vi "Measurement Logic.vi"() -> ()   [LabVIEW 2021, in "Ripple_PMIC.lvlib"]
uses:
  Ripple_PMIC.lvlib
  <vilib>/MeasurementLink/MeasurementLink Measurement Server/Measure Call Context/Measure Call Context.lvclass
  Measurement Results.ctl
  Measurement Configuration.ctl
  <instrlib>/niDCPower/nidcpower.llb/niDCPower Output Function.ctl
  <instrlib>/niDCPower/nidcpower.llb/niDCPower Sense.ctl
  <instrlib>/niDCPower/nidcpower.llb/niDCPower Source Mode.ctl
  <instrlib>/niDCPower/nidcpower.llb/niDCPower Wait For Event - Event.ctl
  <instrlib>/niDCPower/nidcpower.llb/niDCPower Measurement Type.ctl
  <instrlib>/niScope/Controls/niScope vertical coupling.ctl
  <instrlib>/niScope/Controls/niScope trigger slope.ctl
  <instrlib>/niScope/Controls/niScope trigger coupling.ctl
  <instrlib>/niScope/Configure/Trigger/niScope Configure Trigger Edge.vi
  <vilib>/MeasurementLink/MeasurementLink Measurement Server/Measure Call Context/Accessor/Is Canceled.vi
  <instrlib>/niDCPower/nidcpower.llb/niDCPower Get Channel Name From String.vi
  <instrlib>/niScope/Controls/niScope timestamp type.ctl
  <vilib>/measure/NI_MAPro.lvlib
  <vilib>/measure/madcrms.llb/Basic Averaged DC-RMS for 1 Chan.vi
  <instrlib>/niScope/Acquire/Fetch/niScope Fetch WDT.vi
panel:
  in  "measurement configuration":T1={"Mode of operation"=enum."Perform measurement", "Source resource name"="", "Source voltage level"=10.0, "Source current limit"=15.0, "Load resource name"="", "Load current level"=6.0, "Load voltage limit range"=6.0, "Scope resource name"="", "Scope channel name"="0", "Scope sample rate"=10000.0, "Scope acquisition time"=3.0, "Scope probe attenuation"=1.0}
  out "measurement results":T2
  out "measure call context out":refnum<class "Measure Call Context.lvclass">
  in  "measure call context in":refnum<class "Measure Call Context.lvclass">
  out "error out":errorcluster
  in  "error in":errorcluster
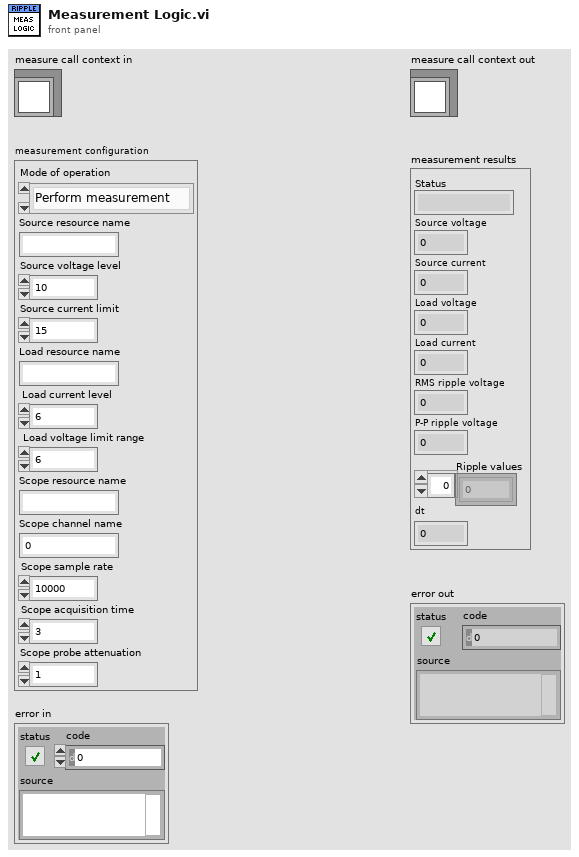
[diagram p1: front panel]
types:
  T1 = typedef "Ripple_PMIC.lvlib/Measurement Configuration.ctl" = cluster{"Mode of operation":enum32{"Power on the DUT", "Perform measurement", "Power off the DUT"}, "Source resource name":string, "Source voltage level":dbl, "Source current limit":dbl, "Load resource name":string, "Load current level":dbl, "Load voltage limit range":dbl, "Scope resource name":string, "Scope channel name":string, "Scope sample rate":dbl, "Scope acquisition time":dbl, "Scope probe attenuation":dbl}
  T2 = typedef "Ripple_PMIC.lvlib/Measurement Results.ctl" = cluster{"Status":string, "Source voltage":dbl, "Source current":dbl, "Load voltage":dbl, "Load current":dbl, "RMS ripple voltage":dbl, "P-P ripple voltage":dbl, "Ripple values":dbl[], "dt":dbl}
  T3 = cluster{"Source Session":refnum<k15>, "Load Session":refnum<k15>, "Scope Session":refnum<k15>, "Source channel":string, "Load channel":string}
  T4 = enum32{"Power on the DUT", "Perform measurement", "Power off the DUT"}
  T5 = typedef "niDCPower Wait For Event - Event.ctl" = i32
  T6 = typedef "niDCPower Source Mode.ctl" = i32
  T7 = typedef "niDCPower Sense.ctl" = i32
  T8 = typedef "niDCPower Output Function.ctl" = i32
  T9 = typedef "niDCPower Measurement Type.ctl" = i32
  T10 = typedef "niScope trigger coupling.ctl" = u16
  T11 = typedef "niScope trigger slope.ctl" = i32
  T12 = typedef "niScope vertical coupling.ctl" = i32
  T13 = typedef "niScope timestamp type.ctl" = i32
  T14 = cluster{"actualSamples":i32, "absoluteInitialX":dbl, "relativeInitialX":dbl, "xIncrement":dbl, "offset":dbl, "gain":dbl, "reserved1":dbl, "reserved2":dbl}
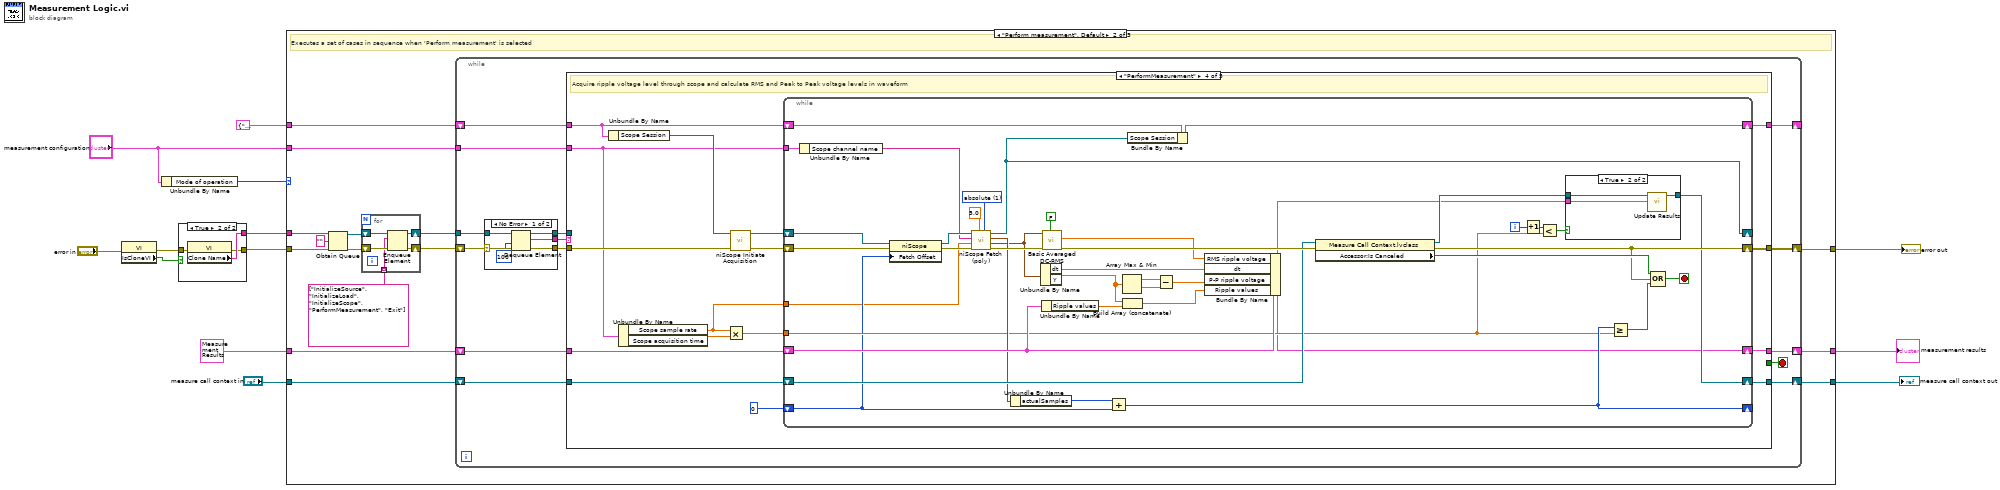
[diagram p0: block diagram]
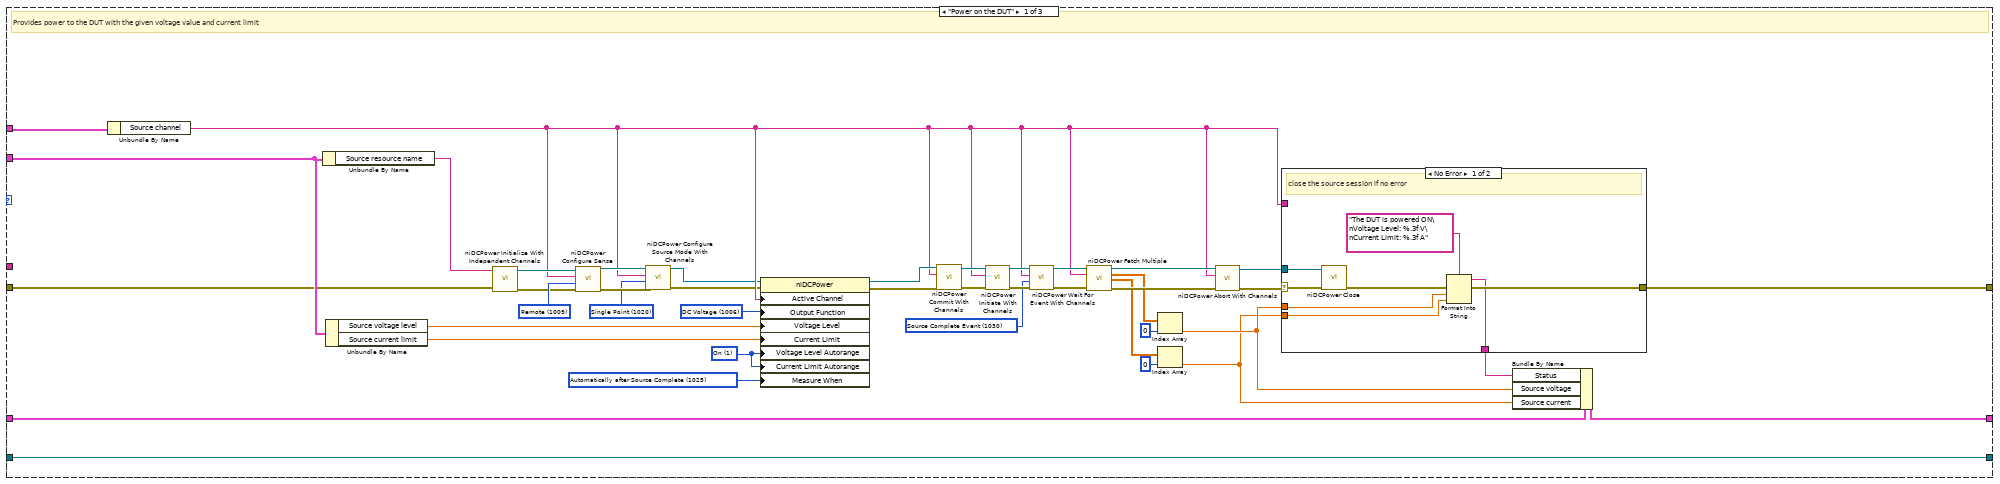
[diagram p2: hidden frame]
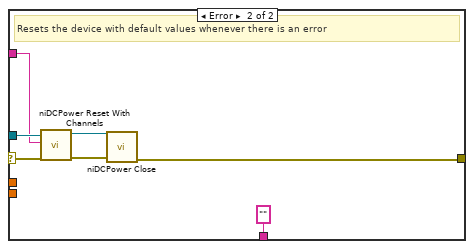
[diagram p3: hidden frame]
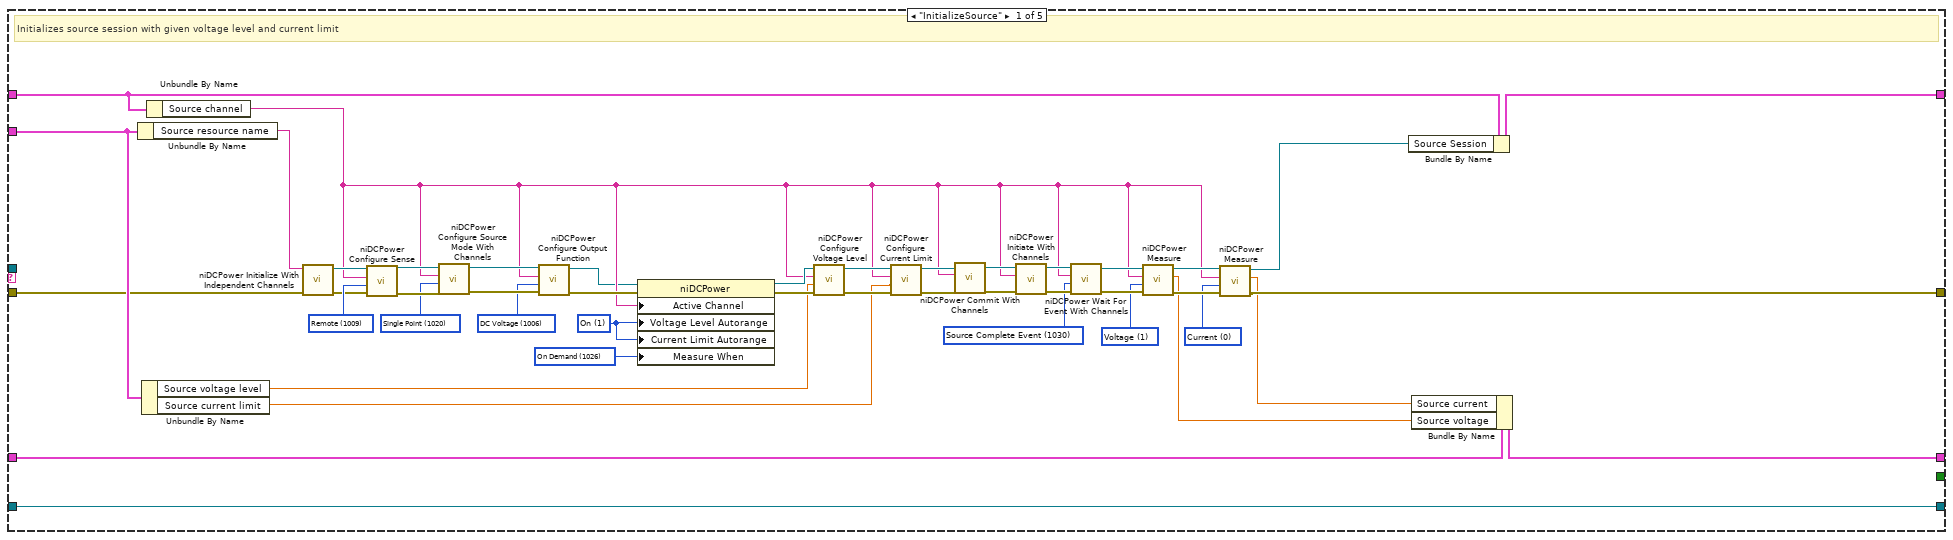
[diagram p4: hidden frame]
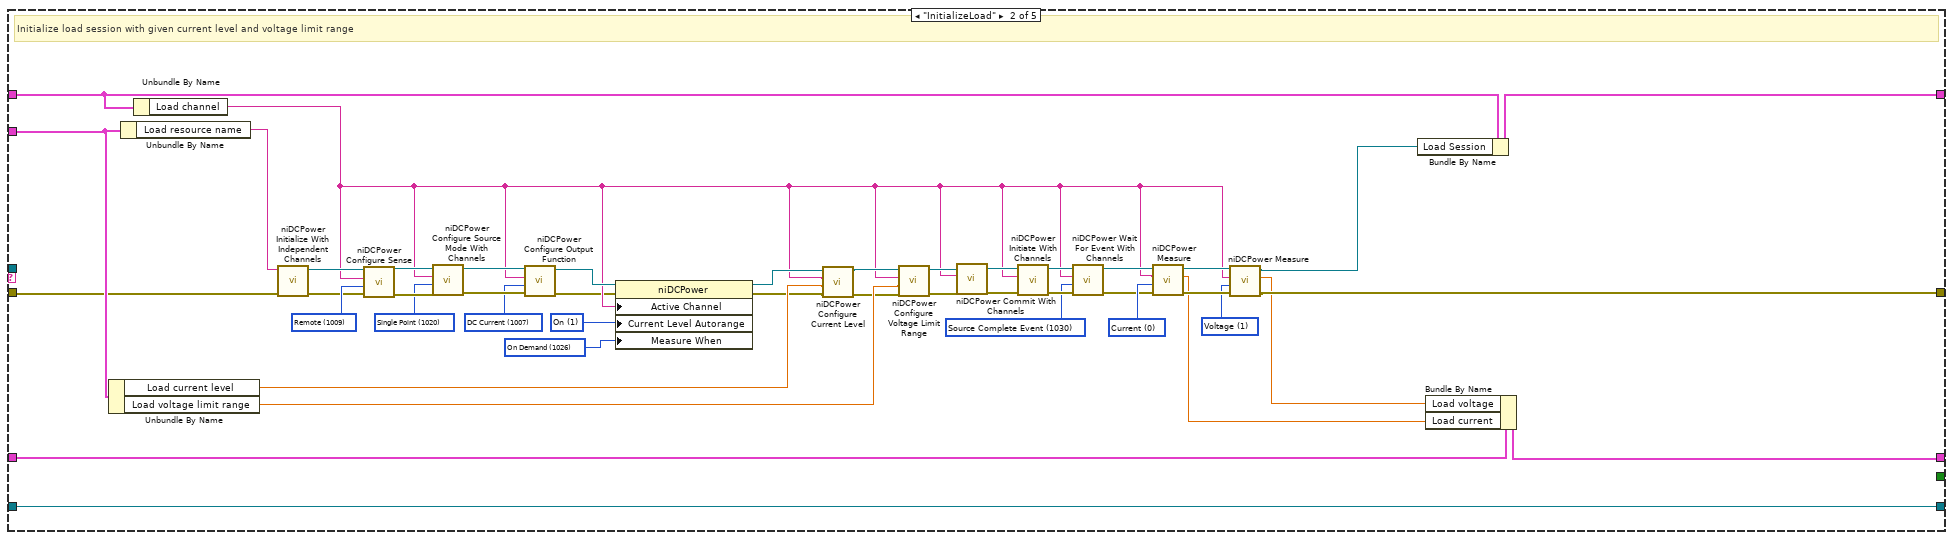
[diagram p5: hidden frame]
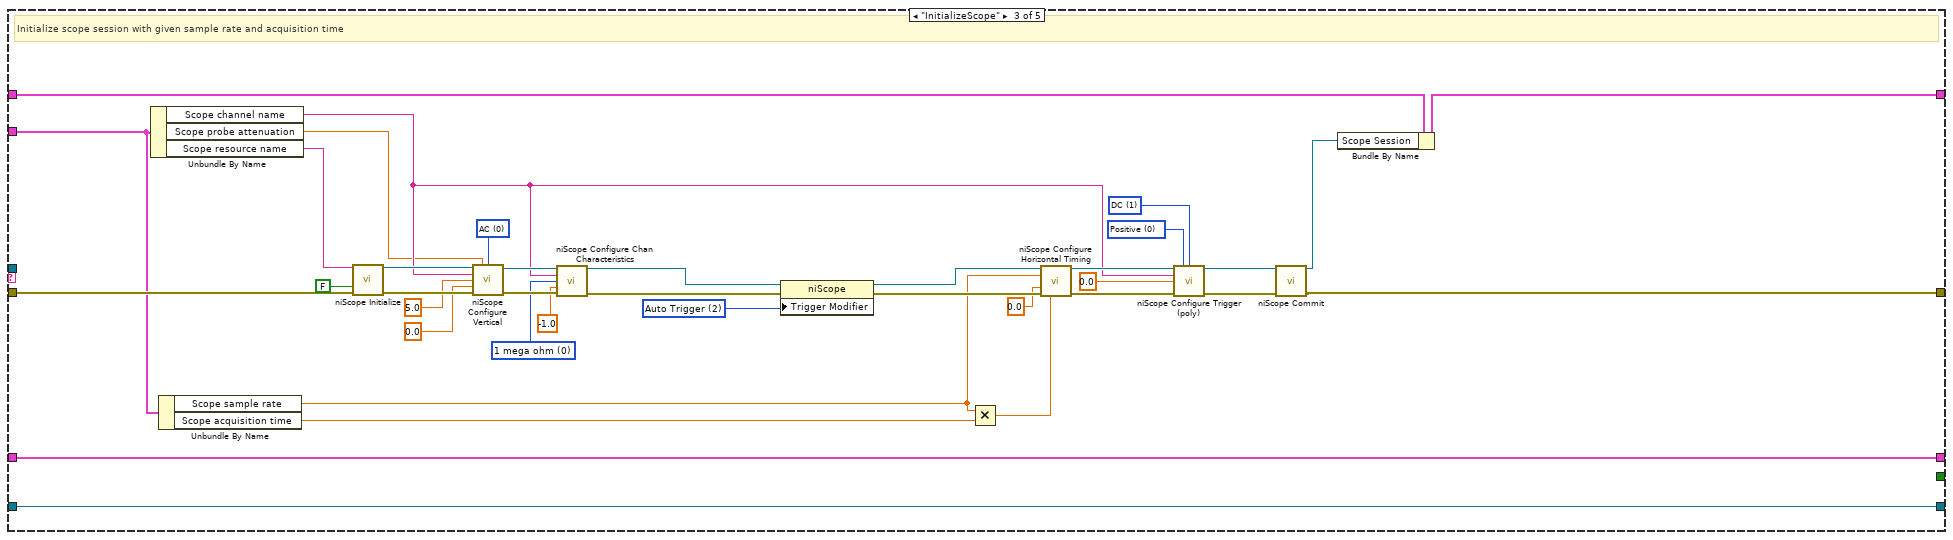
[diagram p6: hidden frame]
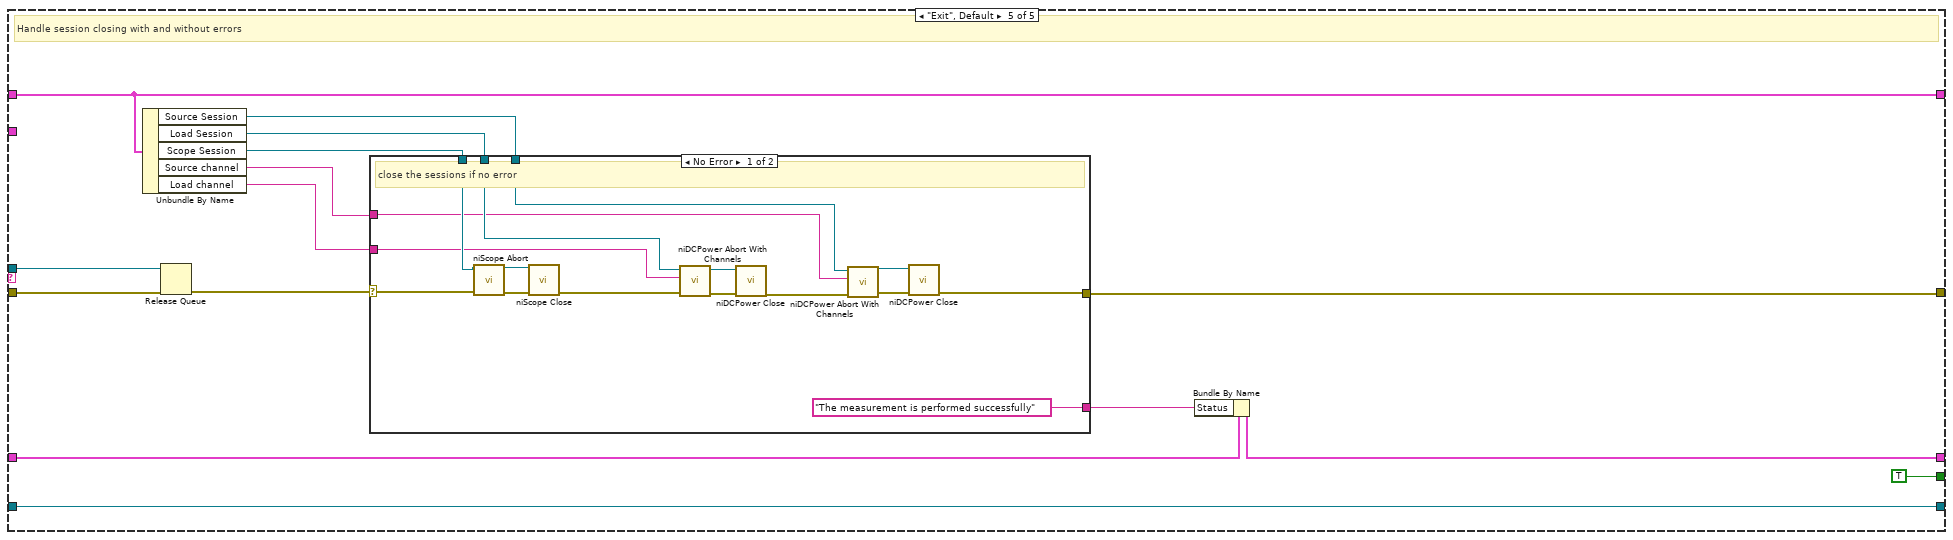
[diagram p8: hidden frame]
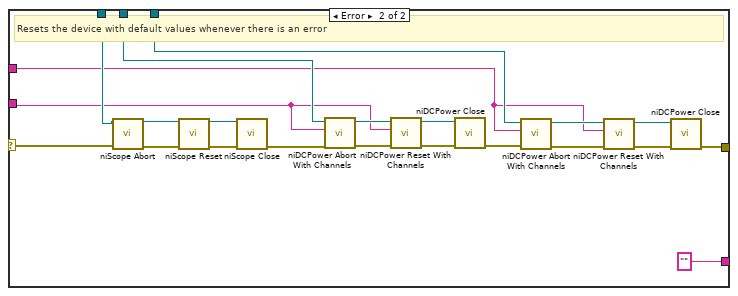
[diagram p9: hidden frame]
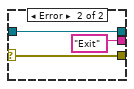
[diagram p10: hidden frame]
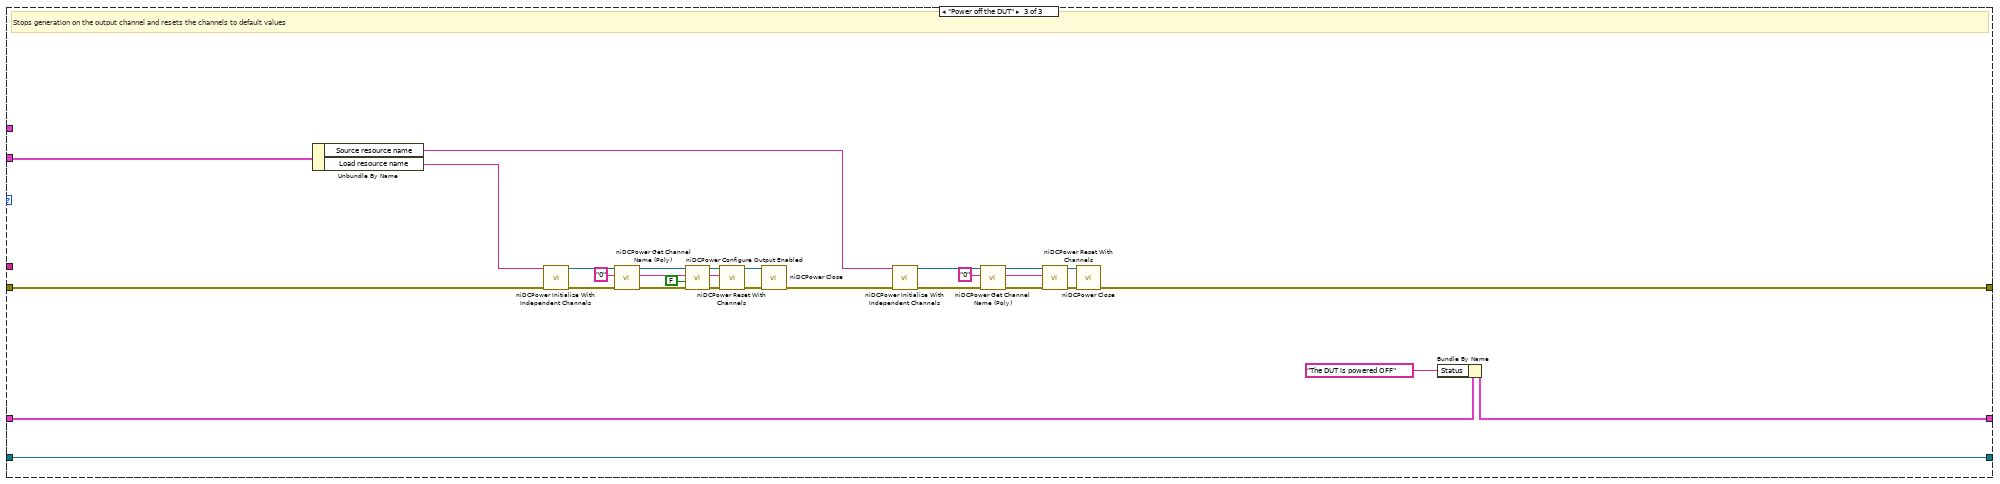
[diagram p11: hidden frame]
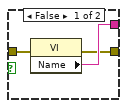
[diagram p12: hidden frame]
diagram:
  n1 = property class="VI"(error in="error in") -> (error out=w12:errorcluster, "IsCloneVI"=w13:bool)  [unwired: 1 in, 1 out]
  n2 = Unbundle By Name("measurement configuration") -> ("Mode of operation"=w6:T4)
  n3 = case shown="True" w13 {
    tunnel: w12 -> [w16 w19]
    tunnel: [w15 w18] -> w4
    tunnel: [w14 w17] -> w5
    frame False {
      n4 = property class="VI"(error in=w16) -> (error out=w14:errorcluster, "Name"=w15:string)  [unwired: 1 in, 1 out]
    }
    frame True {
      n5 = property class="VI"(error in=w19) -> (error out=w17:errorcluster, "Clone Name"=w18:string)  [unwired: 1 in, 1 out]
    }
  }
  n6 = case shown="\"Perform measurement\", Default" w6 {
    tunnel: T3 {"Source Session"="", "Load Session"="", "Scope Session"="", "Source channel"="0", "Load channel"="0"} ("Cluster") -> [w40 w91 _]
    tunnel: T2 {"Status"="", "Source voltage"=0.0, "Source current"=0.0, "Load voltage"=0.0, "Load current"=0.0, "RMS ripple voltage"=0.0, "P-P ripple voltage"=0.0, "Ripple values"=[], "dt"=0.0} ("Measurement Results") -> [w43 w90 w364]
    tunnel: [w38 w89 w368] -> w8
    tunnel: "measurement configuration" -> [w45 w88 w369]
    tunnel: [w44 w87 w363] -> w7
    tunnel: w5 -> [w39 w81 w367]
    tunnel: w4 -> [_ w80 _]
    tunnel: "measure call context in" -> [w21 w78 w361]
    tunnel: [w21 w77 w361] -> w1
    frame "Power on the DUT" {
      w20 = 1025 items=["Automatically after Source Complete"=1025, "On Demand"=1026, "On Measure Trigger"=1027] ("Measurement:Advanced:Measure When")
      w51 = T5 1030 items=["Source Complete Event"=1030, "Measure Complete Event"=1031, "Sequence Iteration Complete Event"=1032, "Sequence Engine Done Event"=1033, "Pulse Complete Event"=1051, "Ready For Pulse Trigger Event"=1052] ("event")
      w25 = 1 items=["Off", "On"] ("Source:DC Voltage:Voltage Level Autorange")
      w58 = T6 1020 items=["Single Point"=1020, "Sequence"=1021] ("source mode")
      w61 = T7 1009 items=["Local"=1008, "Remote"=1009] ("sense")
      w26 = T8 1006 items=["DC Voltage"=1006, "DC Current"=1007, "Pulse Voltage"=1049, "Pulse Current"=1050] ("output function")
      # "Provides power to the DUT with the given voltage value and current limit"
      n7 = Unbundle By Name(w40) -> ("Source channel"=w35:string)
      n8 = Unbundle By Name(w45) -> ("Source resource name"=w50:string)
      n9 = Unbundle By Name(w45) -> ("Source voltage level"=w23:dbl, "Source current limit"=w24:dbl)
      n10 = call <instrlib>:"niDCPower Initialize With Independent Channels.vi"("error in (no error)"=w39, "resource name"=w50) -> ("error out"=w37:errorcluster, "instrument handle out"=w36:refnum<k15>)  [unwired: 8 in]
      n11 = call <instrlib>:"niDCPower Configure Sense.vi"("error in (no error)"=w37, "sense"=w61, "channel name"=w35, "instrument handle"=w36) -> ("error out"=w59:errorcluster, "instrument handle out"=w60:refnum<k15>)  [unwired: 6 in]
      n12 = call <instrlib>:"niDCPower Configure Source Mode With Channels.vi"("error in (no error)"=w59, "source mode"=w58, "channel name"=w35, "instrument handle"=w60) -> ("error out"=w22:errorcluster, "instrument handle out"=w27:refnum<k15>)  [unwired: 6 in]
      n13 = property class="niDCPower"(reference=w27, error in=w22, "Active Channel"=w35, "Output Function"=w26, "Voltage Level"=w23, "Current Limit"=w24, "Voltage Level Autorange"=w25, "Current Limit Autorange"=w25, "Measure When"=w20) -> (reference out=w57:refnum<k15>, error out=w56:errorcluster)
      n14 = call <instrlib>:"niDCPower Commit With Channels.vi"("error in (no error)"=w56, "channel name"=w35, "instrument handle"=w57) -> ("error out"=w54:errorcluster, "instrument handle out"=w55:refnum<k15>)  [unwired: 7 in]
      n15 = call <instrlib>:"niDCPower Initiate With Channels.vi"("error in (no error)"=w54, "channel name"=w35, "instrument handle"=w55) -> ("error out"=w53:errorcluster, "instrument handle out"=w52:refnum<k15>)  [unwired: 7 in]
      n16 = call <instrlib>:"niDCPower Wait For Event With Channels.vi"("error in (no error)"=w53, "event"=w51, "channel name"=w35, "instrument handle"=w52) -> ("error out"=w48:errorcluster, "instrument handle out"=w49:refnum<k15>)  [unwired: 6 in]
      n17 = call <instrlib>:"niDCPower Fetch Multiple.vi"("instrument handle"=w49, "channel name"=w35, "error in (no error)"=w48) -> ("instrument handle out"=w47:refnum<k15>, "voltage measurements"=w34:dbl[], "current measurements"=w33:dbl[], "error out"=w46:errorcluster)  [unwired: 7 in, 2 out]
      n18 = Index Array(array=w34, index=0) -> (element=w30:dbl)
      n19 = Index Array(array=w33, index=0) -> (element=w29:dbl)
      n20 = call <instrlib>:"niDCPower Abort With Channels.vi"("error in (no error)"=w46, "channel name"=w35, "instrument handle"=w47) -> ("error out"=w42:errorcluster, "instrument handle out"=w41:refnum<k15>)  [unwired: 7 in]
      n21 = case shown="No Error" w42 {
        selector: w42 -> [w68 w75]
        tunnel: w41 -> [w69 w76]
        tunnel: [w66 w72] -> w38
        tunnel: w30 -> [w64 _]
        tunnel: w29 -> [w63 _]
        tunnel: [w62 ""] -> w28
        tunnel: w35 -> [_ w70]
        frame No Error {
          # "close the source session if no error"
          n22 = call <instrlib>:"niDCPower Close.vi"("error in (no error)"=w68, "instrument handle"=w69) -> ("error out"=w65:errorcluster)  [unwired: 9 in]
          n23 = Format Into String(format string="The DUT is powered ON\nVoltage Level: %.3f V\nCurrent Limit: %.3f A" ("message"), error in=w65, w64, w63) -> (resulting string=w62:string, error out=w66:errorcluster)  [unwired: 1 in]
        }
        frame Error {
          # "Resets the device with default values whenever there is an error"
          n24 = call <instrlib>:"niDCPower Reset With Channels.vi"("error in (no error)"=w75, "channel name"=w70, "instrument handle"=w76) -> ("error out"=w74:errorcluster, "instrument handle out"=w73:refnum<k15>)  [unwired: 7 in]
          n25 = call <instrlib>:"niDCPower Close.vi"("error in (no error)"=w74, "instrument handle"=w73) -> ("error out"=w72:errorcluster)  [unwired: 9 in]
        }
      }
      n26 = Bundle By Name(cluster=w43, "Status"=w28, "Source voltage"=w30, "Source current"=w29) -> (w44:T2)
    }
    frame "Perform measurement", Default {
      # "Executes a set of cases in sequence when 'Perform measurement' is selected"
      n27 = Obtain Queue(name (unnamed)=w80, element data type="", error in (no error)=w81) -> (queue out=w83:refnum<queue>, error out=w82:errorcluster)  [unwired: 2 in, 1 out]
      n28 = for {
        shift-right: [w94] -> w86
        shift-left: w83 -> [w96]
        shift-right: [w93] -> w85
        shift-left: w82 -> [w95]
        tunnel: string[] ["InitializeSource", "InitializeLoad", "InitializeScope", "PerformMeasurement", "Exit"] ("Step sequence") -> [w92] mode=indexing
        n29 = Enqueue Element(queue=w96, element=w92, error in (no error)=w95) -> (queue out=w94:refnum<queue>, error out=w93:errorcluster)  [unwired: 1 in, 1 out]
      }
      n30 = while {
        tunnel: w88 -> [w107]
        shift-right: [w101] -> _
        shift-left: w91 -> [w102]
        shift-right: [w105] -> w89
        shift-left: w85 -> [w110]
        shift-right: [w103] -> w87
        shift-left: w90 -> [w104]
        tunnel: w86 -> [w109]
        shift-right: [w98] -> w77
        shift-left: w78 -> [w99]
        stop <- w97 stop-if-true
        n31 = case shown="No Error" w110 {
          selector: w110 -> [w355 w359]
          tunnel: w109 -> [w357 w358]
          tunnel: [w356 "Exit" ("t")] -> w108
          tunnel: [w354 w359] -> w106
          tunnel: [w352 w358] -> w100
          frame No Error {
            n32 = Dequeue Element(queue=w357, timeout in ms (-1)=100, error in (no error)=w355) -> (queue out=w352:refnum<queue>, element=w356:string, error out=w354:errorcluster)  [unwired: 1 out]
          }
          frame Error {
          }
        }
        n33 = case shown="\"PerformMeasurement\"" w108 {
          tunnel: w107 -> [w143 w186 w218 w238 _]
          tunnel: w106 -> [w130 w159 w236 w253 w308]
          tunnel: [w119 w165 w205 w245 w310] -> w105
          tunnel: w102 -> [w116 w162 w215 w247 w305]
          tunnel: [w127 w173 w214 w246 w305] -> w101
          tunnel: w104 -> [w118 w164 w210 w243 w302]
          tunnel: [w117 w163 w210 w244 w301] -> w103
          tunnel: [_ _ _ _ TRUE] -> w97
          tunnel: w100 -> [_ _ _ _ w307]
          tunnel: w99 -> [w114 w158 w203 w242 w299]
          tunnel: [w114 w158 w203 w240 w299] -> w98
          frame "InitializeSource" {
            w121 = T9 0 items=["Current", "Voltage"] ("measurement type")
            w122 = T9 1 items=["Current", "Voltage"] ("measurement type")
            w132 = T5 1030 items=["Source Complete Event"=1030, "Measure Complete Event"=1031, "Sequence Iteration Complete Event"=1032, "Sequence Engine Done Event"=1033, "Pulse Complete Event"=1051, "Ready For Pulse Trigger Event"=1052] ("event")
            w146 = 1026 items=["Automatically after Source Complete"=1025, "On Demand"=1026, "On Measure Trigger"=1027] ("Measurement:Advanced:Measure When")
            w147 = 1 items=["Off", "On"] ("Source:DC Voltage:Voltage Level Autorange")
            w152 = T6 1020 items=["Single Point"=1020, "Sequence"=1021] ("source mode")
            w155 = T7 1009 items=["Local"=1008, "Remote"=1009] ("sense")
            w149 = T8 1006 items=["DC Voltage"=1006, "DC Current"=1007, "Pulse Voltage"=1049, "Pulse Current"=1050] ("output function")
            # "Initializes source session with given voltage level and current limit"
            n34 = Unbundle By Name(w143) -> ("Source resource name"=w131:string)
            n35 = Unbundle By Name(w143) -> ("Source voltage level"=w142:dbl, "Source current limit"=w139:dbl)
            n36 = Unbundle By Name(w116) -> ("Source channel"=w115:string)
            n37 = call <instrlib>:"niDCPower Initialize With Independent Channels.vi"("error in (no error)"=w130, "resource name"=w131) -> ("error out"=w128:errorcluster, "instrument handle out"=w129:refnum<k15>)  [unwired: 8 in]
            n38 = call <instrlib>:"niDCPower Configure Sense.vi"("error in (no error)"=w128, "sense"=w155, "channel name"=w115, "instrument handle"=w129) -> ("error out"=w153:errorcluster, "instrument handle out"=w154:refnum<k15>)  [unwired: 6 in]
            n39 = call <instrlib>:"niDCPower Configure Source Mode With Channels.vi"("error in (no error)"=w153, "source mode"=w152, "channel name"=w115, "instrument handle"=w154) -> ("error out"=w150:errorcluster, "instrument handle out"=w151:refnum<k15>)  [unwired: 6 in]
            n40 = call <instrlib>:"niDCPower Configure Output Function.vi"("error in (no error)"=w150, "output function"=w149, "channel name"=w115, "instrument handle"=w151) -> ("error out"=w148:errorcluster, "instrument handle out"=w111:refnum<k15>)  [unwired: 6 in]
            n41 = property class="niDCPower"(reference=w111, error in=w148, "Active Channel"=w115, "Voltage Level Autorange"=w147, "Current Limit Autorange"=w147, "Measure When"=w146) -> (reference out=w145:refnum<k15>, error out=w144:errorcluster)
            n42 = call <instrlib>:"niDCPower Configure Voltage Level.vi"("error in (no error)"=w144, "voltage level"=w142, "channel name"=w115, "instrument handle"=w145) -> ("error out"=w140:errorcluster, "instrument handle out"=w141:refnum<k15>)  [unwired: 6 in]
            n43 = call <instrlib>:"niDCPower Configure Current Limit.vi"("error in (no error)"=w140, "current limit"=w139, "channel name"=w115, "instrument handle"=w141) -> ("error out"=w138:errorcluster, "instrument handle out"=w137:refnum<k15>)  [unwired: 6 in]
            n44 = call <instrlib>:"niDCPower Commit With Channels.vi"("error in (no error)"=w138, "channel name"=w115, "instrument handle"=w137) -> ("error out"=w135:errorcluster, "instrument handle out"=w136:refnum<k15>)  [unwired: 7 in]
            n45 = call <instrlib>:"niDCPower Initiate With Channels.vi"("error in (no error)"=w135, "channel name"=w115, "instrument handle"=w136) -> ("error out"=w134:errorcluster, "instrument handle out"=w133:refnum<k15>)  [unwired: 7 in]
            n46 = call <instrlib>:"niDCPower Wait For Event With Channels.vi"("error in (no error)"=w134, "event"=w132, "channel name"=w115, "instrument handle"=w133) -> ("error out"=w125:errorcluster, "instrument handle out"=w126:refnum<k15>)  [unwired: 6 in]
            n47 = call <instrlib>:"niDCPower Measure.vi"("error in (no error)"=w125, "measurement type"=w122, "channel name"=w115, "instrument handle"=w126) -> ("error out"=w123:errorcluster, "measurement"=w112:dbl, "instrument handle out"=w124:refnum<k15>)  [unwired: 5 in]
            n48 = call <instrlib>:"niDCPower Measure.vi"("error in (no error)"=w123, "measurement type"=w121, "channel name"=w115, "instrument handle"=w124) -> ("error out"=w119:errorcluster, "measurement"=w113:dbl, "instrument handle out"=w120:refnum<k15>)  [unwired: 5 in]
            n49 = Bundle By Name(cluster=w116, "Source Session"=w120) -> (w127:T3)
            n50 = Bundle By Name(cluster=w118, "Source current"=w113, "Source voltage"=w112) -> (w117:T2)
          }
          frame "InitializeLoad" {
            w169 = T9 1 items=["Current", "Voltage"] ("measurement type")
            w170 = T9 0 items=["Current", "Voltage"] ("measurement type")
            w187 = T5 1030 items=["Source Complete Event"=1030, "Measure Complete Event"=1031, "Sequence Iteration Complete Event"=1032, "Sequence Engine Done Event"=1033, "Pulse Complete Event"=1051, "Ready For Pulse Trigger Event"=1052] ("event")
            w192 = 1026 items=["Automatically after Source Complete"=1025, "On Demand"=1026, "On Measure Trigger"=1027] ("Measurement:Advanced:Measure When")
            w193 = 1 items=["Off", "On"] ("Source:DC Voltage:Voltage Level Autorange")
            w197 = T6 1020 items=["Single Point"=1020, "Sequence"=1021] ("source mode")
            w200 = T7 1009 items=["Local"=1008, "Remote"=1009] ("sense")
            w194 = T8 1007 items=["DC Voltage"=1006, "DC Current"=1007, "Pulse Voltage"=1049, "Pulse Current"=1050] ("output function")
            # "Initialize load session with given current level and voltage limit range"
            n51 = Unbundle By Name(w186) -> ("Load current level"=w183:dbl, "Load voltage limit range"=w178:dbl)
            n52 = Unbundle By Name(w186) -> ("Load resource name"=w176:string)
            n53 = Unbundle By Name(w162) -> ("Load channel"=w161:string)
            n54 = call <instrlib>:"niDCPower Initialize With Independent Channels.vi"("error in (no error)"=w159, "resource name"=w176) -> ("error out"=w174:errorcluster, "instrument handle out"=w175:refnum<k15>)  [unwired: 8 in]
            n55 = call <instrlib>:"niDCPower Configure Sense.vi"("error in (no error)"=w174, "sense"=w200, "channel name"=w161, "instrument handle"=w175) -> ("error out"=w198:errorcluster, "instrument handle out"=w199:refnum<k15>)  [unwired: 6 in]
            n56 = call <instrlib>:"niDCPower Configure Source Mode With Channels.vi"("error in (no error)"=w198, "source mode"=w197, "channel name"=w161, "instrument handle"=w199) -> ("error out"=w195:errorcluster, "instrument handle out"=w196:refnum<k15>)  [unwired: 6 in]
            n57 = call <instrlib>:"niDCPower Configure Output Function.vi"("error in (no error)"=w195, "output function"=w194, "channel name"=w161, "instrument handle"=w196) -> ("error out"=w160:errorcluster, "instrument handle out"=w185:refnum<k15>)  [unwired: 6 in]
            n58 = property class="niDCPower"(reference=w185, error in=w160, "Active Channel"=w161, "Current Level Autorange"=w193, "Measure When"=w192) -> (reference out=w184:refnum<k15>, error out=w182:errorcluster)
            n59 = call <instrlib>:"niDCPower Configure Current Level.vi"("error in (no error)"=w182, "current level"=w183, "channel name"=w161, "instrument handle"=w184) -> ("error out"=w177:errorcluster, "instrument handle out"=w179:refnum<k15>)  [unwired: 6 in]
            n60 = call <instrlib>:"niDCPower Configure Voltage Limit Range.vi"("error in (no error)"=w177, "voltage limit range"=w178, "channel name"=w161, "instrument handle"=w179) -> ("error out"=w181:errorcluster, "instrument handle out"=w180:refnum<k15>)  [unwired: 6 in]
            n61 = call <instrlib>:"niDCPower Commit With Channels.vi"("error in (no error)"=w181, "channel name"=w161, "instrument handle"=w180) -> ("error out"=w190:errorcluster, "instrument handle out"=w191:refnum<k15>)  [unwired: 7 in]
            n62 = call <instrlib>:"niDCPower Initiate With Channels.vi"("error in (no error)"=w190, "channel name"=w161, "instrument handle"=w191) -> ("error out"=w189:errorcluster, "instrument handle out"=w188:refnum<k15>)  [unwired: 7 in]
            n63 = call <instrlib>:"niDCPower Wait For Event With Channels.vi"("error in (no error)"=w189, "event"=w187, "channel name"=w161, "instrument handle"=w188) -> ("error out"=w167:errorcluster, "instrument handle out"=w168:refnum<k15>)  [unwired: 6 in]
            n64 = call <instrlib>:"niDCPower Measure.vi"("error in (no error)"=w167, "measurement type"=w170, "channel name"=w161, "instrument handle"=w168) -> ("error out"=w171:errorcluster, "measurement"=w157:dbl, "instrument handle out"=w172:refnum<k15>)  [unwired: 5 in]
            n65 = call <instrlib>:"niDCPower Measure.vi"("error in (no error)"=w171, "measurement type"=w169, "channel name"=w161, "instrument handle"=w172) -> ("error out"=w165:errorcluster, "measurement"=w156:dbl, "instrument handle out"=w166:refnum<k15>)  [unwired: 5 in]
            n66 = Bundle By Name(cluster=w162, "Load Session"=w166) -> (w173:T3)
            n67 = Bundle By Name(cluster=w164, "Load voltage"=w156, "Load current"=w157) -> (w163:T2)
          }
          frame "InitializeScope" {
            w223 = T10 1 items=["AC"=0, "DC"=1, "HF Reject"=3, "LF Reject"=4, "AC Plus HF Reject"=1001] ("trigger coupling")
            w204 = T11 0 items=["Positive", "Negative"] ("trigger slope")
            w224 = 2 items=["None"=1, "Auto Trigger"=2] ("Triggering:Trigger Modifier")
            w228 = u32 0 items=["1 mega ohm"=0, "50 ohms"=2] ("input impedance")
            w231 = T12 0 items=["AC", "DC", "Ground"] ("vertical coupling")
            # "Initialize scope session with given sample rate and acquisition time"
            n68 = Unbundle By Name(w218) -> ("Scope channel name"=w209:string, "Scope probe attenuation"=w202:dbl, "Scope resource name"=w201:string)
            n69 = Unbundle By Name(w218) -> ("Scope sample rate"=w208:dbl, "Scope acquisition time"=w207:dbl)
            n70 = call <instrlib>:"niScope Initialize.vi"("resource name"=w201, "reset device"=FALSE, "error in"=w236) -> ("instrument handle"=w235:refnum<k15>, "error out"=w234:errorcluster)  [unwired: 11 in]
            n71 = call <instrlib>:"niScope Configure Vertical.vi"("instrument handle"=w235, "probe attenuation"=w202, "vertical coupling"=w231, "channels"=w209, "vertical range"=5.0, "vertical offset"=0.0, "error in"=w234) -> ("instrument handle out"=w230:refnum<k15>, "error out"=w229:errorcluster)  [unwired: 7 in]
            n72 = call <instrlib>:"niScope Configure Chan Characteristics.vi"("instrument handle"=w230, "channels"=w209, "input impedance"=w228, "maximum input frequency"=-1.0, "error in"=w229) -> ("instrument handle out"=w226:refnum<k15>, "error out"=w225:errorcluster)  [unwired: 9 in]
            n73 = property class="niScope"(reference=w226, error in=w225, "Trigger Modifier"=w224) -> (reference out=w222:refnum<k15>, error out=w221:errorcluster)
            n74 = Multiply(x=w208, y=w207) -> (x*y=w206:dbl)
            n75 = call <instrlib>:"niScope Configure Horizontal Timing.vi"("instrument handle"=w222, "min sample rate"=w208, "reference position"=0.0, "error in"=w221, "min record length"=w206) -> ("instrument handle out"=w220:refnum<k15>, "error out"=w219:errorcluster)  [unwired: 9 in]
            n76 = call-poly <instrlib>:"niScope Configure Trigger (poly).vi"("instrument handle"=w220, "trigger slope"=w204, "trigger coupling"=w223, "trigger source"=w209, "trigger level"=0.0, "error in"=w219) -> ("instrument handle out"=w213:refnum<k15>, "error out"=w212:errorcluster)  [unwired: 8 in]
            n77 = call <instrlib>:"niScope Commit.vi"("instrument handle"=w213, "error in"=w212) -> ("instrument handle out"=w211:refnum<k15>, "error out"=w205:errorcluster)  [unwired: 12 in]
            n78 = Bundle By Name(cluster=w215, "Scope Session"=w211) -> (w214:T3)
          }
          frame "PerformMeasurement" {
            # "Acquire ripple voltage level through scope and calculate RMS and Peak to Peak voltage levels in waveform"
            n79 = Unbundle By Name(w247) -> ("Scope Session"=w252:refnum<k15>)
            n80 = Unbundle By Name(w238) -> ("Scope sample rate"=w239:dbl, "Scope acquisition time"=w249:dbl)
            n81 = Multiply(x=w239, y=w249) -> (x*y=w248:dbl)
            n82 = call <instrlib>:"niScope Initiate Acquisition.vi"("instrument handle"=w252, "error in"=w253) -> ("instrument handle out"=w250:refnum<k15>, "error out"=w251:errorcluster)  [unwired: 12 in]
            n83 = while {
              shift-right: [w287] -> w245
              shift-left: w251 -> [w271]
              shift-right: [w255] -> w244
              shift-left: w243 -> [w279]
              shift-right: [w293] -> w246
              shift-left: w247 -> [w289]
              shift-right: [w283] -> w240
              shift-left: w242 -> [w285]
              tunnel: w248 -> [w274]
              shift-right: [w254] -> _
              shift-left: w250 -> [w272]
              shift-right: [w275] -> _
              shift-left: 0 -> [w273]
              tunnel: w239 -> [w267]
              tunnel: w238 -> [w260]
              i -> [w281]
              stop <- w264 stop-if-true
              w294 = T13 1 items=["relative", "absolute"] ("timestamp Type")
              n84 = Unbundle By Name(w260) -> ("Scope channel name"=w259:string)
              n85 = property class="niScope"(reference=w272, error in=w271, "Fetch Offset"=w273) -> (reference out=w269:refnum<k15>, error out=w270:errorcluster)
              n86 = call-poly <instrlib>:"niScope Fetch (poly).vi"("timestamp Type"=w294, "timeout"=5.0 ("y"), "error in"=w270, "numSamples"=w267, "channels"=w259, "instrument handle"=w269) -> ("error out"=w292:errorcluster, "wfm"=w268:waveform(dbl), "wfm info"=w278:T14, "instrument handle out"=w254:refnum<k15>)  [unwired: 2 in]
              n87 = Unbundle By Name(w278) -> ("actualSamples"=w277:i32)
              n88 = Unbundle By Name(w268) -> ("dt"=w257:dbl, "Y"=w258:dbl[])
              n89 = Unbundle By Name(w279) -> ("Ripple values"=w265:dbl[])
              n90 = call-poly <vilib>:"Basic Averaged DC-RMS.vi"("reset"=FALSE, "error in (no error)"=w292, "signal in"=w268) -> ("error out"=w286:errorcluster, "RMS value"=w256:dbl)  [unwired: 5 in, 2 out]
              n91 = Add(x=w277, y=w273) -> (x+y=w275:i32)
              n92 = Array Max & Min(array=w258) -> (max value=w263:dbl, min value=w262:dbl)  [unwired: 2 out]
              n93 = Build Array (concatenate)(w258, w265) -> (w261:dbl[])
              n94 = Bundle By Name(cluster=w289, "Scope Session"=w254) -> (w293:T3)
              n95 = Subtract(x=w263, y=w262) -> (x-y=w291:dbl)
              n96 = Bundle By Name(cluster=w279, "RMS ripple voltage"=w256, "dt"=w257, "P-P ripple voltage"=w291, "Ripple values"=w261) -> (w255:T2)
              n97 = property class="Measure Call Context.lvclass"(reference=w285, error in=w286) -> (reference out=w284:refnum<class "Measure Call Context.lvclass">, error out=w287:errorcluster, "Accessor:Is Canceled"=w288:bool)
              n98 = Increment(x=w281) -> (x+1=w282:i32)
              n99 = Less?(x=w282, y=w274) -> (x < y?=w280:bool)
              n100 = case shown="True" w280 {
                tunnel: [w295 w298] -> w283
                tunnel: w284 -> [w295 w297]
                tunnel: w255 -> [_ w296]
                frame False {
                }
                frame True {
                  n101 = call <vilib>:"Update Results.vi"("measurement results"=w296, "measure call context in"=w297) -> ("measure call context out"=w298:refnum<class "Measure Call Context.lvclass">)  [unwired: 8 in, 1 out]
                }
              }
              n102 = Greater Or Equal?(x=w275, y=w274) -> (x >= y?=w276:bool)
              n103 = Compound Arithmetic op=OR(w288, w287, w276) -> (w264:bool)
            }
          }
          frame "Exit", Default {
            # "Handle session closing with and without errors"
            n104 = Unbundle By Name(w305) -> ("Source Session"=w313:refnum<k15>, "Load Session"=w312:refnum<k15>, "Scope Session"=w311:refnum<k15>, "Source channel"=w304:string, "Load channel"=w303:string)
            n105 = Release Queue(queue=w307, error in (no error)=w308) -> (error out=w306:errorcluster)  [unwired: 1 in, 2 out]
            n106 = case shown="No Error" w306 {
              selector: w306 -> [w322 w350]
              tunnel: w313 -> [w314 w332]
              tunnel: w312 -> [w318 w333]
              tunnel: w311 -> [w329 w351]
              tunnel: [w317 w335] -> w310
              tunnel: w304 -> [w315 w330]
              tunnel: w303 -> [w321 w331]
              tunnel: ["The measurement is performed successfully" ("Status") "" ("Status")] -> w300
              frame No Error {
                # "close the sessions if no error"
                n107 = call <instrlib>:"niScope Abort.vi"("instrument handle"=w329, "error in"=w322) -> ("instrument handle out"=w326:refnum<k15>, "error out"=w325:errorcluster)  [unwired: 12 in]
                n108 = call <instrlib>:"niScope Close.vi"("instrument handle"=w326, "error in"=w325) -> ("error out"=w319:errorcluster)  [unwired: 13 in]
                n109 = call <instrlib>:"niDCPower Abort With Channels.vi"("error in (no error)"=w319, "channel name"=w321, "instrument handle"=w318) -> ("error out"=w323:errorcluster, "instrument handle out"=w324:refnum<k15>)  [unwired: 7 in]
                n110 = call <instrlib>:"niDCPower Close.vi"("error in (no error)"=w323, "instrument handle"=w324) -> ("error out"=w316:errorcluster)  [unwired: 9 in]
                n111 = call <instrlib>:"niDCPower Abort With Channels.vi"("error in (no error)"=w316, "channel name"=w315, "instrument handle"=w314) -> ("error out"=w327:errorcluster, "instrument handle out"=w328:refnum<k15>)  [unwired: 7 in]
                n112 = call <instrlib>:"niDCPower Close.vi"("error in (no error)"=w327, "instrument handle"=w328) -> ("error out"=w317:errorcluster)  [unwired: 9 in]
              }
              frame Error {
                # "Resets the device with default values whenever there is an error"
                n113 = call <instrlib>:"niScope Abort.vi"("instrument handle"=w351, "error in"=w350) -> ("instrument handle out"=w341:refnum<k15>, "error out"=w340:errorcluster)  [unwired: 12 in]
                n114 = call <instrlib>:"niScope Reset.vi"("instrument handle"=w341, "error in"=w340) -> ("instrument handle out"=w339:refnum<k15>, "error out"=w338:errorcluster)  [unwired: 12 in]
                n115 = call <instrlib>:"niScope Close.vi"("instrument handle"=w339, "error in"=w338) -> ("error out"=w336:errorcluster)  [unwired: 13 in]
                n116 = call <instrlib>:"niDCPower Abort With Channels.vi"("error in (no error)"=w336, "channel name"=w331, "instrument handle"=w333) -> ("error out"=w344:errorcluster, "instrument handle out"=w345:refnum<k15>)  [unwired: 7 in]
                n117 = call <instrlib>:"niDCPower Reset With Channels.vi"("error in (no error)"=w344, "channel name"=w331, "instrument handle"=w345) -> ("error out"=w343:errorcluster, "instrument handle out"=w342:refnum<k15>)  [unwired: 7 in]
                n118 = call <instrlib>:"niDCPower Close.vi"("error in (no error)"=w343, "instrument handle"=w342) -> ("error out"=w334:errorcluster)  [unwired: 9 in]
                n119 = call <instrlib>:"niDCPower Abort With Channels.vi"("error in (no error)"=w334, "channel name"=w330, "instrument handle"=w332) -> ("error out"=w347:errorcluster, "instrument handle out"=w349:refnum<k15>)  [unwired: 7 in]
                n120 = call <instrlib>:"niDCPower Reset With Channels.vi"("error in (no error)"=w347, "channel name"=w330, "instrument handle"=w349) -> ("error out"=w346:errorcluster, "instrument handle out"=w348:refnum<k15>)  [unwired: 7 in]
                n121 = call <instrlib>:"niDCPower Close.vi"("error in (no error)"=w346, "instrument handle"=w348) -> ("error out"=w335:errorcluster)  [unwired: 9 in]
              }
            }
            n122 = Bundle By Name(cluster=w302, "Status"=w300) -> (w301:T2)
          }
        }
      }
    }
    frame "Power off the DUT" {
      # "Stops generation on the output channel and resets the channels to default values"
      n123 = Unbundle By Name(w369) -> ("Source resource name"=w371:string, "Load resource name"=w374:string)
      n124 = call <instrlib>:"niDCPower Initialize With Independent Channels.vi"("error in (no error)"=w367, "resource name"=w374) -> ("error out"=w375:errorcluster, "instrument handle out"=w373:refnum<k15>)  [unwired: 8 in]
      n125 = call-poly <instrlib>:"niDCPower Get Channel Name (Poly).vi"("error in (no error)"=w375, "index"="0", "instrument handle"=w373) -> ("error out"=w382:errorcluster, "name"=w380:string, "instrument handle out"=w381:refnum<k15>)  [unwired: 6 in]
      n126 = call <instrlib>:"niDCPower Configure Output Enabled.vi"("error in (no error)"=w382, "output enabled"=FALSE, "channel name"=w380, "instrument handle"=w381) -> ("error out"=w389:errorcluster, "instrument handle out"=w388:refnum<k15>)  [unwired: 6 in]
      n127 = call <instrlib>:"niDCPower Reset With Channels.vi"("error in (no error)"=w389, "channel name"=w380, "instrument handle"=w388) -> ("error out"=w383:errorcluster, "instrument handle out"=w384:refnum<k15>)  [unwired: 7 in]
      n128 = call <instrlib>:"niDCPower Close.vi"("error in (no error)"=w383, "instrument handle"=w384) -> ("error out"=w378:errorcluster)  [unwired: 9 out]
      n129 = call <instrlib>:"niDCPower Initialize With Independent Channels.vi"("error in (no error)"=w378, "resource name"=w371) -> ("error out"=w372:errorcluster, "instrument handle out"=w370:refnum<k15>)  [unwired: 8 in]
      n130 = call-poly <instrlib>:"niDCPower Get Channel Name (Poly).vi"("error in (no error)"=w372, "index"="0", "instrument handle"=w370) -> ("error out"=w377:errorcluster, "name"=w376:string, "instrument handle out"=w379:refnum<k15>)  [unwired: 6 in]
      n131 = call <instrlib>:"niDCPower Reset With Channels.vi"("error in (no error)"=w377, "channel name"=w376, "instrument handle"=w379) -> ("error out"=w386:errorcluster, "instrument handle out"=w385:refnum<k15>)  [unwired: 7 in]
      n132 = call <instrlib>:"niDCPower Close.vi"("error in (no error)"=w386, "instrument handle"=w385) -> ("error out"=w368:errorcluster)  [unwired: 9 out]
      n133 = Bundle By Name(cluster=w364, "Status"="The DUT is powered OFF") -> (w363:T2)
    }
  }
  "error out" <- w8
  "measure call context out" <- w1
  "measurement results" <- w7
